vi "Teleop.vi"(10 "Match Info":T1={"Autonomous Elapsed Seconds"=0.0, "TeleOp Elapsed Seconds"=0.0, "Disabled Elapsed Seconds"=0.0, "Visited Autonomous"=FALSE, "Visited TeleOp"=FALSE, "Visited Disabled"=FALSE, "Autonomous Settings"={"Autonomous Style"=enum."Independent", "VI Refnum"=refnum}}, 11 "Call Context":T2) -> ()   [LabVIEW 2015]
doc: "This VI is called for each TeleOp packet received from the DS where the robot is not disabled. It is often used to read from the joysticks and update I/O or to update setpoints for timed control loops. It should complete and return within 20 milliseconds or it may miss DS packets."
uses:
  <vilib>/Rock Robotics/WPI/DriverStation/WPI_DriverStationDerivedRobotMode.ctl
  <vilib>/Rock Robotics/WPI/DriverStation/WPI_DriverStationMatch Info.ctl
  <vilib>/Rock Robotics/WPI/Utilities/WPI_GetSetVariantRefNum.vi
  <vilib>/Rock Robotics/Network Tables/NT Write Boolean Array.vi
  <vilib>/Rock Robotics/Network Tables/NT Write Numeric Array.vi
  <vilib>/Rock Robotics/Network Tables/NT Read Boolean.vi
  <vilib>/Rock Robotics/Network Tables/NT Read Number.vi
  <vilib>/Rock Robotics/WPI/Relay/WPI_RelayValue.ctl
panel:
  out "Sample Slider 0":dbl(slide) scale=0.0..5.0
  out "Sample Boolean 1":bool
  out "Sample Boolean 0":bool
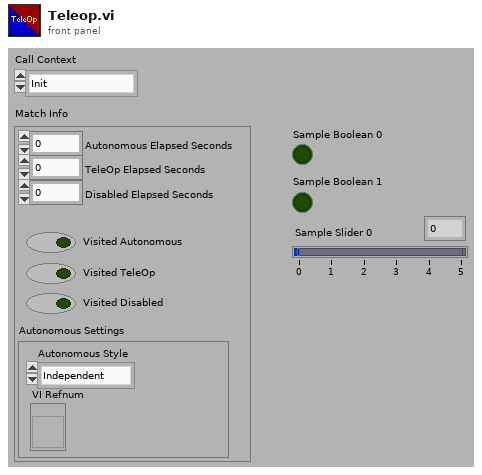
[diagram p1: front panel]
types:
  T1 = typedef "WPI_DriverStationMatch Info.ctl" = cluster{"Autonomous Elapsed Seconds":dbl, "TeleOp Elapsed Seconds":dbl, "Disabled Elapsed Seconds":dbl, "Visited Autonomous":bool, "Visited TeleOp":bool, "Visited Disabled":bool, "Autonomous Settings":cluster{"Autonomous Style":enum16{"Iterative", "Independent"}, "VI Refnum":refnum<vi>}}
  T2 = typedef "WPI_DriverStationDerivedRobotMode.ctl" = enum16{"Init", "Execute", "Stop"}
  T3 = typedef "WPI_JoystickDevRef.ctl" = cluster{"Device":T4}
  T4 = typedef "WPI_JoystickDeviceEnum.ctl" = enum16{"USB 0", "USB 1", "USB 2", "USB 3", "USB 4", "USB 5"}
  T5 = typedef "WPI_MotorControlDeviceRef.ctl" = cluster{"DeviceStatus":errorcluster, "Type":T6, "PWM":cluster{"PWM Channel":T7, "DeadBand":T8}, "CAN":cluster{"Device Number":u8, "Control Mode":T9, "Semaphore":T10, "Max Vout":dbl, "TalonSRX Control Mode":T11}, "Invert":bool}
  T6 = typedef "WPI_MotorControlType.ctl" = enum16{"PWM", "CAN", "CANTalonSRX"}
  T7 = typedef "FPGA_DIOPWMChannel.ctl" = enum8{"PWM 0", "PWM 1", "PWM 2", "PWM 3", "PWM 4", "PWM 5", "PWM 6", "PWM 7", "PWM 8", "PWM 9", "PWM MXP 0", "PWM MXP 1", "PWM MXP 2", "PWM MXP 3", "PWM MXP 4", "PWM MXP 5", "PWM MXP 6", "PWM MXP 7", "PWM MXP 8", "PWM MXP 9", "Invalid"}
  T8 = typedef "WPI_PWMDeadband.ctl" = cluster{"Name":string, "maxPositivePwm":i32, "minPositivePwm":i32, "centerPwm":i32, "maxNegativePwm":i32, "minNegativePwm":i32, "angularRange":u16}
  T9 = typedef "WPI_CANJaguar_ControlMode.ctl" = enum8{"Percent VBus", "Current", "Speed", "Position", "Voltage"}
  T10 = typedef "Semaphore RefNum" = refnum<k1>
  T11 = typedef "WPI_CANTalonSRX_APIControlMode.ctl" = enum8{"Percent VBus", "Speed", "Position", "Slave", "Unchanged / Invalid", "Voltage Compensation", "Current", "Motion Profile"}
  T12 = typedef "WPI_RelayValue.ctl" = enum16{"Off", "On", "Forward", "Reverse"}
  T13 = typedef "WPI_RelayDevRef.ctl" = cluster{"DevStatus":errorcluster, "Relay Channel":T14, "Relay Direction":T15}
  T14 = typedef "FPGA_DIORelayChannel.ctl" = enum8{"Relay 0", "Relay 1", "Relay 2", "Relay 3", "Invalid"}
  T15 = typedef "WPI_RelayDirection.ctl" = enum16{"Both directions", "Forward only", "Reverse only"}
  T16 = typedef "WPI_RobotDriveDevRef.ctl" = cluster{"DevStatus":errorcluster, "Motors[]":T5[], "Square Inputs":bool, "Max Output":dbl}
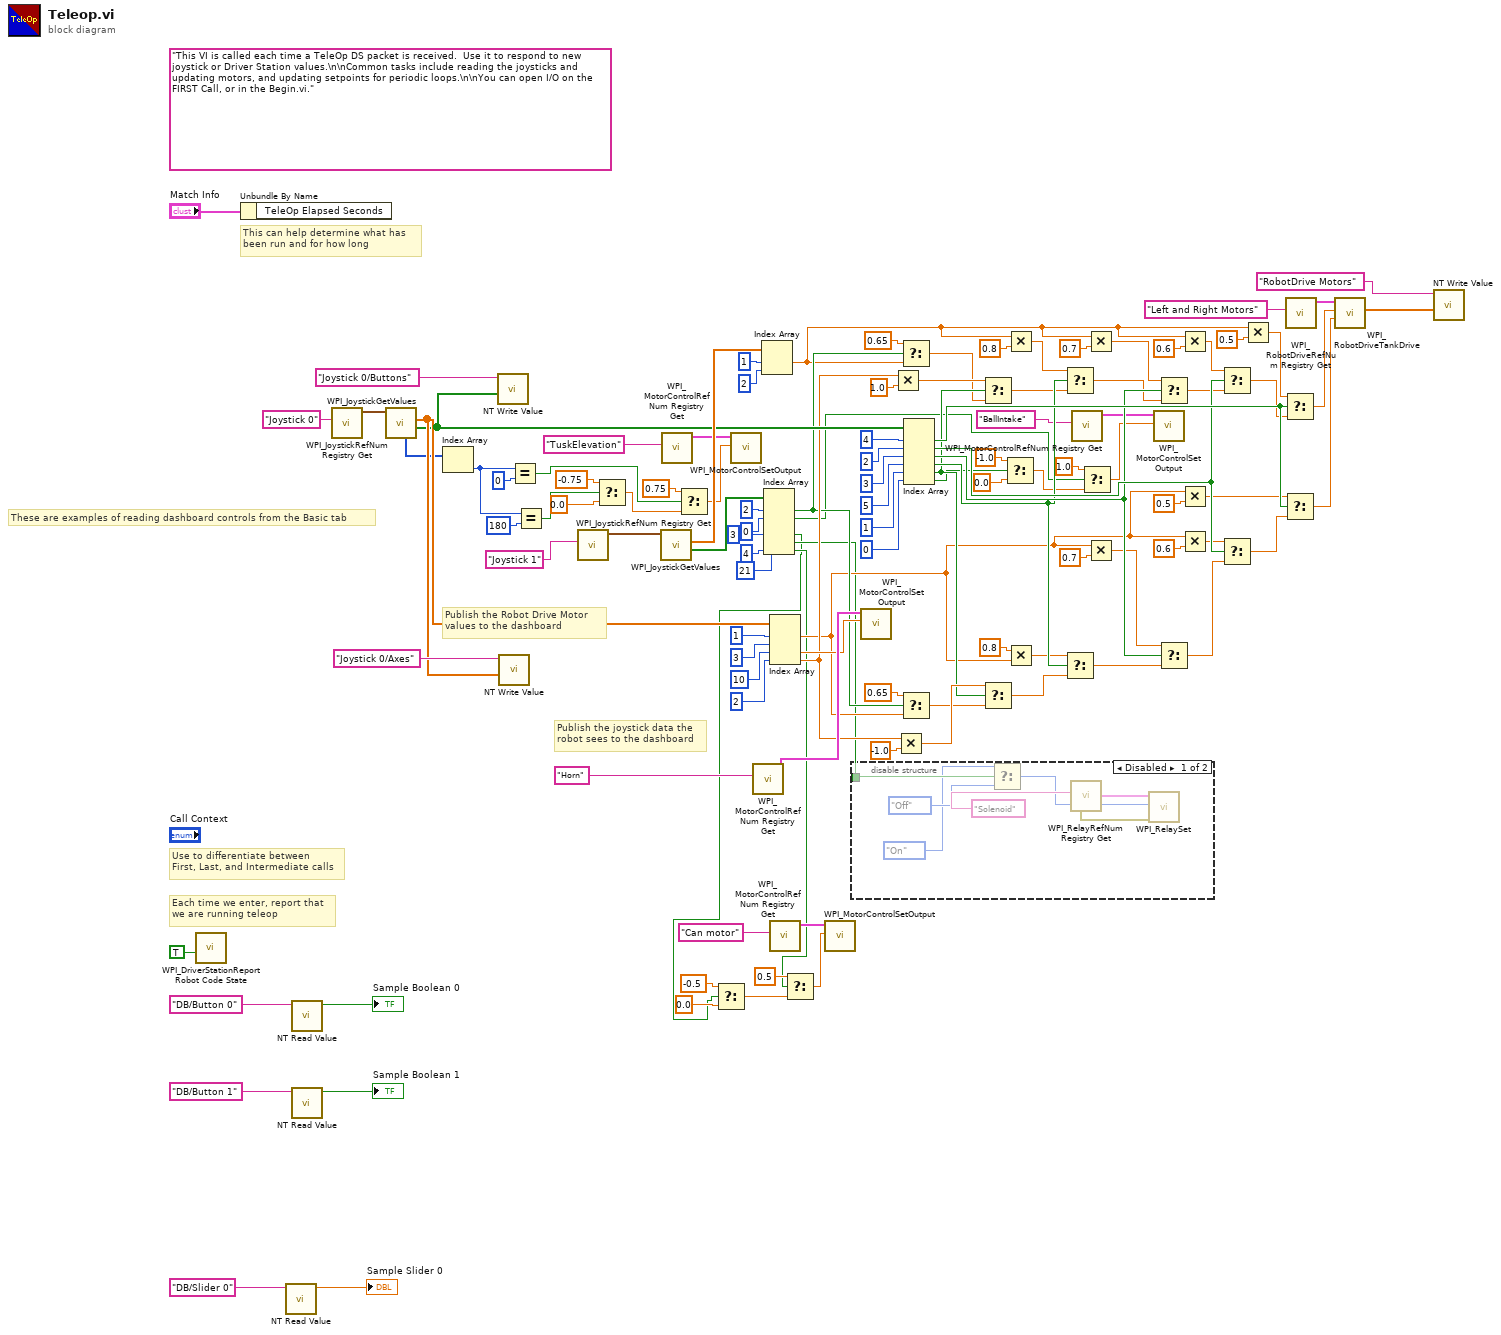
[diagram p0: block diagram]
diagram:
  (unwired) "This VI is called each time a TeleOp DS packet is received.  Use it to respond to new joystick or Driver Station values.\n\nCommon tasks include reading the joysticks and updating motors, and updating setpoints for periodic loops.\n\nYou can open I/O on the FIRST Call, or in the Begin.vi."
  # "These are examples of reading dashboard controls from the Basic tab"
  # "Publish the Robot Drive Motor\nvalues to the dashboard"
  # "Publish the joystick data the\nrobot sees to the dashboard"
  # "Each time we enter, report that\nwe are running teleop"
  # "Use to differentiate between\nFirst, Last, and Intermediate calls"
  # "This can help determine what has\nbeen run and for how long"
  n1 = call <vilib>:"WPI_DriverStationReport Robot Code State.vi"("TeleOp"=TRUE ("Autonomous")) -> ()  [unwired: 10 in, 1 out]
  n2 = Unbundle By Name("Match Info") -> ()  [unwired: 1 out]
  n3 = call-poly <vilib>:"NT Read Value.vi"("Name"="DB/Slider 0" ("refnum name")) -> ("Numeric"=→"Sample Slider 0":dbl)  [unwired: 9 in, 1 out]
  n4 = call-poly <vilib>:"NT Read Value.vi"("Name"="DB/Button 0" ("refnum name")) -> ("Boolean"=→"Sample Boolean 0":bool)  [unwired: 9 in, 1 out]
  n5 = call-poly <vilib>:"NT Read Value.vi"("Name"="DB/Button 1" ("refnum name")) -> ("Boolean"=→"Sample Boolean 1":bool)  [unwired: 9 in, 1 out]
  n6 = call <vilib>:"WPI_JoystickRefNum Registry Get.vi"("refnum name"="Joystick 0") -> ("JoystickDevRef"=w114:T3)  [unwired: 1 in, 9 out]
  n7 = call <vilib>:"WPI_JoystickGetValues.vi"("JoystickDevRef"=w114) -> ("Buttons"=w57:bool[], "Axes"=w110:dbl[], "POVs"=w15:i16[])  [unwired: 6 in, 2 out]
  n8 = Index Array(array=w15) -> (element=w14:i16)  [unwired: 1 in]
  n9 = call-poly <vilib>:"NT Write Value.vi"("Boolean Array"=w57, "Name"="Joystick 0/Buttons") -> ()  [unwired: 9 in, 1 out]
  n10 = call-poly <vilib>:"NT Write Value.vi"("Numeric Array"=w110, "Name"="Joystick 0/Axes") -> ()  [unwired: 9 in, 1 out]
  n11 = Equal?(x=w14, y=i16 0) -> (x = y?=w27:bool)
  n12 = Equal?(x=w14, y=i16 180) -> (x = y?=w28:bool)
  n13 = call <vilib>:"WPI_JoystickRefNum Registry Get.vi"("refnum name"="Joystick 1") -> ("JoystickDevRef"=w96:T3)  [unwired: 1 in, 9 out]
  n14 = Select(t=-0.75, s=w28, f=0.0) -> (s? t:f=w24:dbl)
  n15 = call <vilib>:"WPI_JoystickGetValues.vi"("JoystickDevRef"=w96) -> ("Buttons"=w56:bool[], "Axes"=w94:dbl[])  [unwired: 6 in, 3 out]
  n16 = call <vilib>:"WPI_MotorControlRefNum Registry Get.vi"("refnum name"="TuskElevation") -> ("MotorControlDevRef"=w35:T5)  [unwired: 9 in, 1 out]
  n17 = Select(t=0.75, s=w27, f=w24) -> (s? t:f=w23:dbl)
  n18 = call <vilib>:"WPI_MotorControlSetOutput.vi"("Output"=w23, "MotorControlDevRef"=w35) -> ()  [unwired: 7 in, 3 out]
  n19 = call <vilib>:"WPI_MotorControlRefNum Registry Get.vi"("refnum name"="Horn") -> ("MotorControlDevRef"=w101:T5)  [unwired: 9 in, 1 out]
  n20 = Index Array(array=w94, index #1=1 ("index"), index #2=2 ("index")) -> (element #1=w40:dbl)  [unwired: 1 out]
  n21 = Index Array(array=w56, index #1=2 ("index"), index #2=0 ("index"), index #4=3 ("index"), index #5=21 ("index"), index #6=4 ("index")) -> (element #1=w43:bool, element #2=w19:bool, element #4=w1:bool, element #5=w13:bool, element #6=w3:bool)  [unwired: 1 in, 1 out]
  n22 = Select(t=-0.5, s=w1, f=0.0) -> (s? t:f=w8:dbl)
  n23 = Index Array(array=w110, index #1=1 ("index"), index #2=3 ("index"), index #3=10 ("index"), index #4=2 ("index")) -> (element #1=w38:dbl, element #3=w100:dbl, element #4=w55:dbl)  [unwired: 1 out]
  n24 = call <vilib>:"WPI_MotorControlRefNum Registry Get.vi"("refnum name"="Can motor") -> ("MotorControlDevRef"=w11:T5)  [unwired: 9 in, 1 out]
  n25 = Select(t=0.5, s=w3, f=w8) -> (s? t:f=w10:dbl)
  n26 = call <vilib>:"WPI_MotorControlSetOutput.vi"("Output"=w10, "MotorControlDevRef"=w11) -> ()  [unwired: 7 in, 3 out]
  n27 = disable-structure shown="Disabled" {
    disable-tunnel: w13 -> [w119 _]
    frame Disabled {
      n28 = Select(t=WPI_RelayValue."On" ("RelayValue"), s=w119, f=WPI_RelayValue."Off" ("RelayValue")) -> (s? t:f=w121:T12)
      n29 = call <vilib>:"WPI_RelayRefNum Registry Get.vi"("refnum name"="Solenoid") -> ("error out"=w123:errorcluster, "RelayDevRef"=w122:T13)  [unwired: 9 in]
      n30 = call <vilib>:"WPI_RelaySet.vi"("error in (no error)"=w123, "RelayValue"=w121, "RelayDevRef"=w122) -> ()  [unwired: 7 in, 2 out]
    }
    frame Enabled {
    }
  }
  n31 = call <vilib>:"WPI_MotorControlSetOutput.vi"("Output"=w100, "MotorControlDevRef"=w101) -> ()  [unwired: 7 in, 3 out]
  n32 = Multiply(x=w55, y=1.0) -> (x*y=w53:dbl)
  n33 = Multiply(x=w55, y=-1.0) -> (x*y=w54:dbl)
  n34 = Select(t=0.65, s=w43, f=w40) -> (s? t:f=w41:dbl)
  n35 = Select(t=0.65, s=w43, f=w38) -> (s? t:f=w39:dbl)
  n36 = Index Array(array=w57, index #1=4 ("index"), index #2=2 ("index"), index #3=3 ("index"), index #4=5 ("index"), index #5=1 ("index"), index #6=0 ("index")) -> (element #1=w87:bool, element #2=w86:bool, element #3=w85:bool, element #4=w84:bool, element #5=w48:bool, element #6=w16:bool)
  n37 = Select(t=w53, s=w48, f=w41) -> (s? t:f=w49:dbl)
  n38 = Select(t=w54, s=w48, f=w39) -> (s? t:f=w50:dbl)
  n39 = Select(t=-1.0, s=w16, f=0.0) -> (s? t:f=w31:dbl)
  n40 = Multiply(x=w40, y=0.8 ("t")) -> (x*y=w59:dbl)
  n41 = Multiply(x=0.8 ("t"), y=w38) -> (x*y=w58:dbl)
  n42 = Select(t=w59, s=w84, f=w49) -> (s? t:f=w69:dbl)
  n43 = Select(t=w58, s=w84, f=w50) -> (s? t:f=w76:dbl)
  n44 = call <vilib>:"WPI_MotorControlRefNum Registry Get.vi"("refnum name"="BallIntake") -> ("MotorControlDevRef"=w34:T5)  [unwired: 9 in, 1 out]
  n45 = Select(t=1.0, s=w19, f=w31) -> (s? t:f=w30:dbl)
  n46 = Multiply(x=w40, y=0.7 ("t")) -> (x*y=w68:dbl)
  n47 = Multiply(x=w38, y=0.7 ("t")) -> (x*y=w75:dbl)
  n48 = call <vilib>:"WPI_MotorControlSetOutput.vi"("Output"=w30, "MotorControlDevRef"=w34) -> ()  [unwired: 7 in, 3 out]
  n49 = Select(t=w68, s=w85, f=w69) -> (s? t:f=w70:dbl)
  n50 = Select(t=w75, s=w85, f=w76) -> (s? t:f=w77:dbl)
  n51 = Multiply(x=w40, y=0.6 ("t")) -> (x*y=w66:dbl)
  n52 = Multiply(x=w38, y=0.5) -> (x*y=w79:dbl)
  n53 = Multiply(x=w38, y=0.6 ("t")) -> (x*y=w73:dbl)
  n54 = Select(t=w66, s=w86, f=w70) -> (s? t:f=w64:dbl)
  n55 = Select(t=w73, s=w86, f=w77) -> (s? t:f=w78:dbl)
  n56 = Multiply(x=w40, y=0.5) -> (x*y=w63:dbl)
  n57 = Select(t=w63, s=w87, f=w64) -> (s? t:f=w82:dbl)
  n58 = Select(t=w79, s=w87, f=w78) -> (s? t:f=w83:dbl)
  n59 = call <vilib>:"WPI_RobotDriveRefNum Registry Get.vi"("refnum name"="Left and Right Motors") -> ("RobotDriveDevRef"=w97:T16)  [unwired: 1 in, 9 out]
  n60 = call <vilib>:"WPI_RobotDriveTankDrive.vi"("Right axis value"=w83, "Left axis value"=w82, "RobotDriveDevRef"=w97) -> ("Motor Values"=w98:dbl[])  [unwired: 6 in, 2 out]
  n61 = call-poly <vilib>:"NT Write Value.vi"("Numeric Array"=w98, "Name"="RobotDrive Motors") -> ()  [unwired: 9 in, 1 out]
